vi "FPSTPS.vi"(9 "Ticks Per Rev":dbl, 10 "Wheel Radius(inches)":dbl, 11 "Feet Per Second":dbl) -> (0 "ticks/sec":dbl, 1 "rev/sec":dbl, 2 "rev/ft":dbl, 3 "rev/in":dbl)   [LabVIEW 2014]
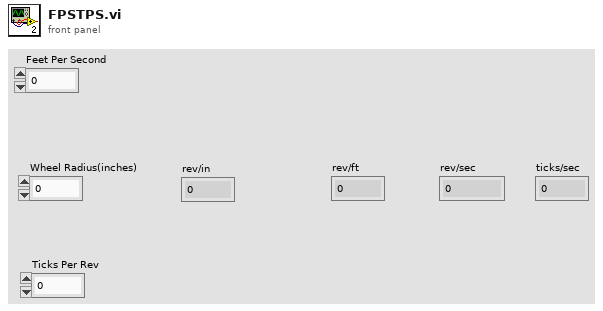
[diagram p1: front panel]
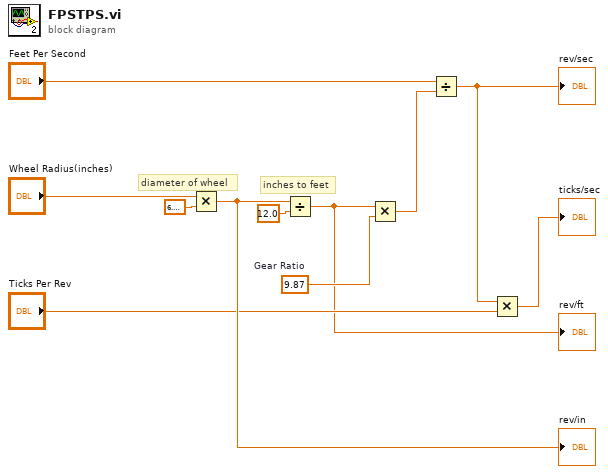
[diagram p0: block diagram]
diagram:
  w4 = 9.87  # Gear Ratio
  # "diameter of wheel"
  # "inches to feet"
  n1 = Multiply(x="Wheel Radius(inches)", y=6.283185307179586) -> (x*y=w9:dbl)
  "rev/in" <- w9
  n2 = Divide(x=w9, y=12.0) -> (x/y=w2:dbl)
  "rev/ft" <- w2
  n3 = Multiply(x=w2, y=w4) -> (x*y=w1:dbl)
  n4 = Divide(x="Feet Per Second", y=w1) -> (x/y=w7:dbl)
  "rev/sec" <- w7
  n5 = Multiply(x=w7, y="Ticks Per Rev") -> (x*y=→"ticks/sec":dbl)
